vi "MISC Fix Mininum Integer Value.vi"(0 "Number":i32, 1 "Min (0)":i32) -> (6 "Max of Number and Min":i32)   [LabVIEW 2011]
doc: "This routine converts a 1-D U32 Hexidecimal Array into a string list. The delimiter may be one or more characters."
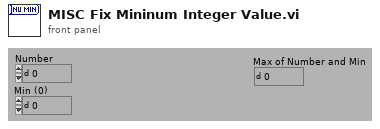
[diagram p1: front panel]
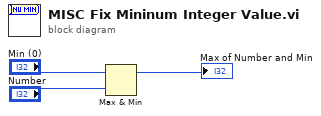
[diagram p0: block diagram]
diagram:
  n1 = Max & Min(x="Min (0)", y="Number") -> (max(x,y)=→"Max of Number and Min":i32)  [unwired: 1 out]
